vi "Sum Waveform Array.vi"(8 "Error In":errorcluster, 9 "Waveform Array":waveform(dbl)[](array[waveform])) -> (0 "Error Out":errorcluster, 1 "Summed Waveform Array":waveform(dbl))   [LabVIEW 2020]
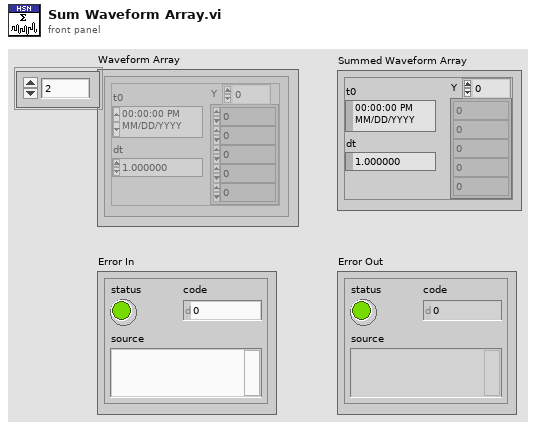
[diagram p1: front panel]
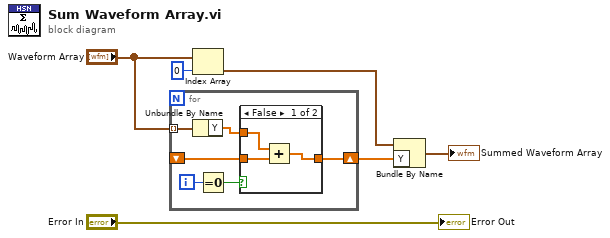
[diagram p0: block diagram]
diagram:
  n1 = for {
    tunnel: "Waveform Array" -> [w7] mode=indexing
    shift-right: [w9] -> w6
    shift-left: _ -> [w8]
    i -> [w11]
    n2 = Unbundle By Name(w7) -> ("Y"=w10:dbl[])
    n3 = Equal To 0?(x=w11) -> (x = 0?=w12:bool)
    n4 = case shown="False" w12 {
      tunnel: w8 -> [w15 _]
      tunnel: [w14 w16] -> w9
      tunnel: w10 -> [w13 w16]
      frame False {
        n5 = Add(x=w13, y=w15) -> (x+y=w14:dbl[])
      }
      frame True {
      }
    }
  }
  n6 = Index Array(array="Waveform Array", index=0) -> (element=w2:waveform(dbl))
  n7 = Bundle By Name(cluster=w2, "Y"=w6) -> (→"Summed Waveform Array":waveform(dbl))
  "Error Out" <- "Error In"
